vi "DG535.set delays.vi"(0 "i ref in":refnum<vi>, 1 "A=":i32(slide) scale=0.0..3.0, 2 "A":dbl min=0.0 max=999.999999999995 format="%.12f", 3 "B=":i32(slide) scale=0.0..3.0, 4 "B":dbl min=0.0 max=999.999999999995 format="%.12f", 5 "error in (no error)":errorcluster, 6 "D=":i32(slide) scale=0.0..3.0, 7 "C=":i32(slide) scale=0.0..3.0, 8 "D":dbl min=0.0 max=999.999999999995 format="%.12f", 9 "C":dbl min=0.0 max=999.999999999995 format="%.12f") -> (14 "i ref out":refnum<vi>, 19 "error out":errorcluster)   [LabVIEW 2014, in "DG535.lvlib"]
doc: "This vi can be used to defined the 4 delays (A, B, C and D) in one shot, by defining a reference channel and a time offset for each channels. One channel must have T0 as a reference."
uses:
  DG535.lvlib
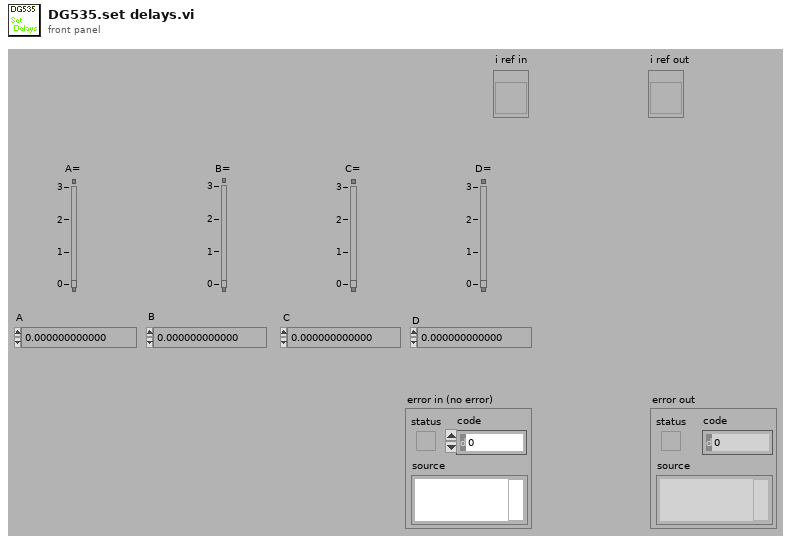
[diagram p1: front panel]
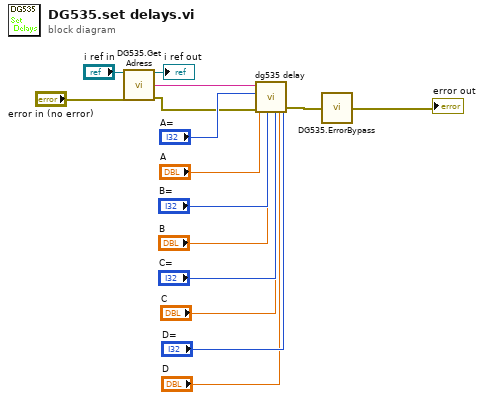
[diagram p0: block diagram]
diagram:
  n1 = call "DG535.Get Adress.vi"("i ref in"="i ref in", "error in (no error)"="error in (no error)") -> ("i ref out"=→"i ref out":refnum<vi>, "address"=w12:string, "error out"=w9:errorcluster)  [unwired: 10 in, 1 out]
  n2 = call "dg535 delay.vi"("C"="C", "D"="D", "D="="D=", "C="="C=", "B"="B", "error in"=w9, "A"="A", "B="="B=", "A="="A=", "GPIB address"=w12) -> ("error out"=w2:errorcluster)
  n3 = call "DG535.ErrorBypass.vi"("error in (no error)"=w2) -> ("error out"=→"error out":errorcluster)  [unwired: 14 in]
